vi "Get Intensity Graph Y Label.vi"(8 "error in (no error)":errorcluster, 11 "graph_utilities in":refnum<class "graph_utilities.lvclass">) -> (0 "error out":errorcluster, 2 "Y Label":string, 3 "graph_utilities out":refnum<class "graph_utilities.lvclass">)   [LabVIEW 2019, in "graph_utilities.lvclass"]
doc: "Get the Y Label of the Intensity Graph"
uses:
  graph_utilities.lvclass
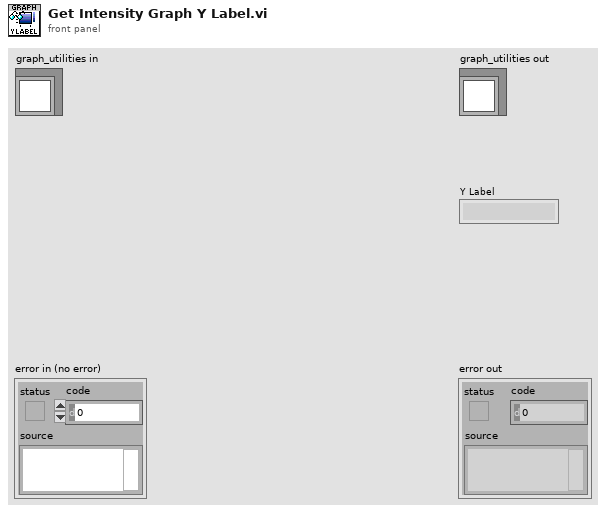
[diagram p1: front panel]
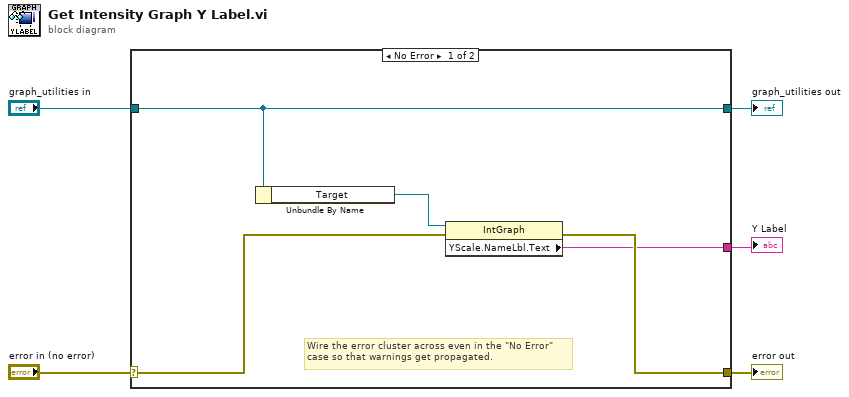
[diagram p0: block diagram]
diagram:
  n1 = case shown="No Error" "error in (no error)" {
    selector: "error in (no error)" -> [w8 w12]
    tunnel: [w7 w12] -> w4
    tunnel: [w10 w11] -> w2
    tunnel: "graph_utilities in" -> [w10 w11]
    tunnel: [w6 _] -> w1
    frame No Error {
      # "Wire the error cluster across even in the \"No Error\"\ncase so that warnings get propagated."
      n2 = Unbundle By Name(w10) -> ("Target"=w9:refnum<vi>)
      n3 = property on="Property Node" class="IntGraph"(reference=w9, error in=w8) -> (error out=w7:errorcluster, "YScale.NameLbl.Text"=w6:string)  [unwired: 1 out]
    }
    frame Error {
    }
  }
  "error out" <- w4
  "graph_utilities out" <- w2
  "Y Label" <- w1
